vi "move_pipes.vi"(8 "error in (no error)":errorcluster, 9 "Y-values":dbl[](array[numeric]), 10 "New Y-value":dbl) -> (0 "error out":errorcluster, 1 "Y-values Out":dbl[](array[numeric]))   [LabVIEW 2019, in "Flappy Bird.lvlib"]
uses:
  Flappy Bird.lvlib
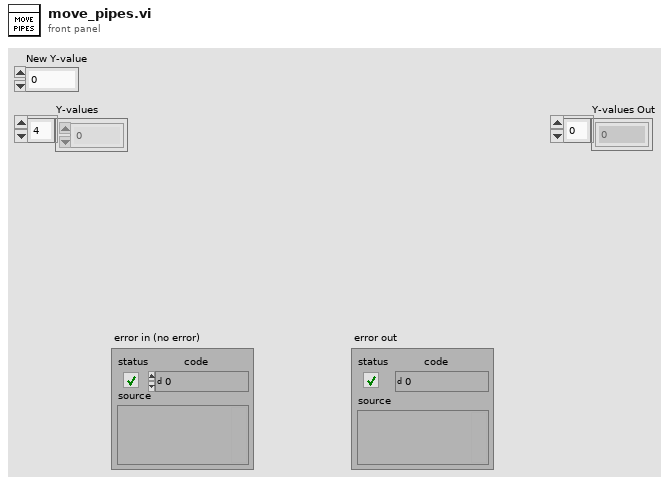
[diagram p1: front panel]
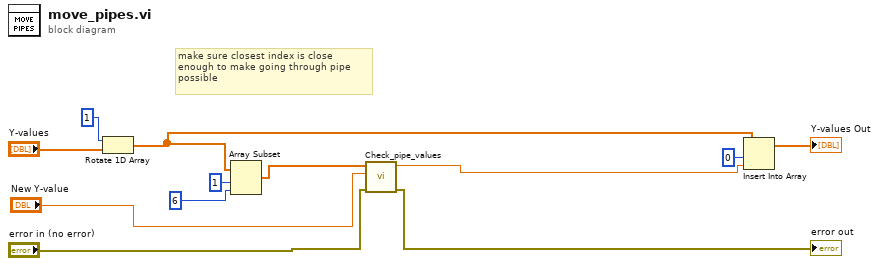
[diagram p0: block diagram]
diagram:
  # "make sure closest index is close\nenough to make going through pipe\npossible"
  n1 = Rotate 1D Array(1:"Y-values", 2:1 ("n")) -> (0:w2:dbl[])
  n2 = Array Subset(array=w2, index=1, length=6) -> (w1:dbl[])
  n3 = call "Check_pipe_values.vi"("error in (no error)"="error in (no error)", "New Y-value in"="New Y-value", "Y-values"=w1) -> ("error out"=→"error out":errorcluster, "New Y-value out"=w7:dbl)  [unwired: 7 in]
  n4 = Insert Into Array(array=w2, index=0, new element=w7) -> (→"Y-values Out":dbl[])
